vi "PDCRecordStatus.vi"(11 "PDCRecordStatus":T2) -> (1 "Color[4]":cluster{u32, u32}[](array[cluster]), 2 "String[4]":string[](array[string]), 3 "Disabled":T1(ring))   [LabVIEW 2015]
uses:
  TypeDefs/PDCRecordStatus.ctl
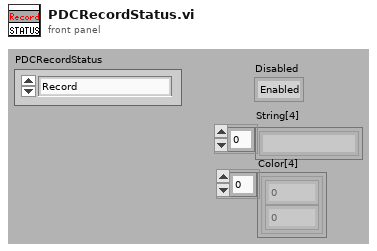
[diagram p1: front panel]
types:
  T1 = enum8{"Enabled", "Disabled", "Disabled and Grayed Out"}
  T2 = typedef "PDCRecordStatus.ctl" = enum16{"Record", "WaitingTRG", "Endless", "Recording"}
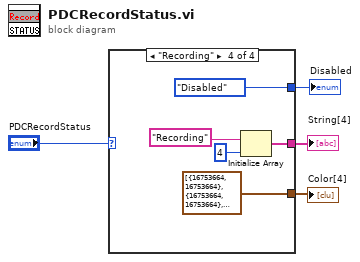
[diagram p0: block diagram]
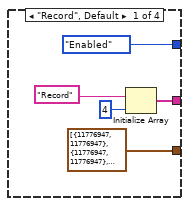
[diagram p2: hidden frame]
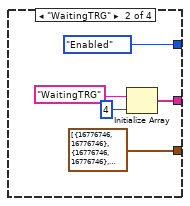
[diagram p3: hidden frame]
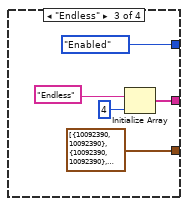
[diagram p4: hidden frame]
diagram:
  n1 = case shown="\"Recording\"" "PDCRecordStatus" {
    tunnel: [w7 w12 w17 w22] -> w4
    tunnel: [cluster{u32, u32}[] [{11776947, 11776947}, {11776947, 11776947}, {8355711, 8355711}, {8355711, 8355711}] ("カラー[4]") cluster{u32, u32}[] [{16776746, 16776746}, {16776746, 16776746}, {8355711, 8355711}, {8355711, 8355711}] ("カラー[4]") cluster{u32, u32}[] [{10092390, 10092390}, {10092390, 10092390}, {8355711, 8355711}, {8355711, 8355711}] ("カラー[4]") cluster{u32, u32}[] [{16753664, 16753664}, {16753664, 16753664}, {8355711, 8355711}, {8355711, 8355711}] ("カラー[4]")] -> w3
    tunnel: [T1."Enabled" ("Disabled") T1."Enabled" ("Disabled") T1."Enabled" ("Disabled") T1."Disabled" ("Disabled")] -> w1
    frame "Record", Default {
      n2 = Initialize Array("Record", 4 ("次元サイズ")) -> (w7:string[])
    }
    frame "WaitingTRG" {
      n3 = Initialize Array("WaitingTRG", 4 ("次元サイズ")) -> (w12:string[])
    }
    frame "Endless" {
      n4 = Initialize Array("Endless", 4 ("次元サイズ")) -> (w17:string[])
    }
    frame "Recording" {
      n5 = Initialize Array("Recording", 4 ("次元サイズ")) -> (w22:string[])
    }
  }
  "String[4]" <- w4
  "Color[4]" <- w3
  "Disabled" <- w1
